vi "joysticki.vi"(9 "Multicolumn Listbox":i32(listbox), 10 "stop":bool) -> (11 "Numeric":i32)   [LabVIEW 2015]
uses:
  <vilib>/MakerHub/Xbox-One-Controller/Private/Type Defs/Xbox Controller Device.ctl
  <vilib>/Utility/inputDevices.llb/closeJoystick.vi
  <vilib>/MakerHub/Xbox-One-Controller/LMH-Xbox-One-Controller.lvlib
panel:
  out "output cluster":T1
  out "mouse info":T2(array[cluster])
  out "key info":T3(array[cluster])
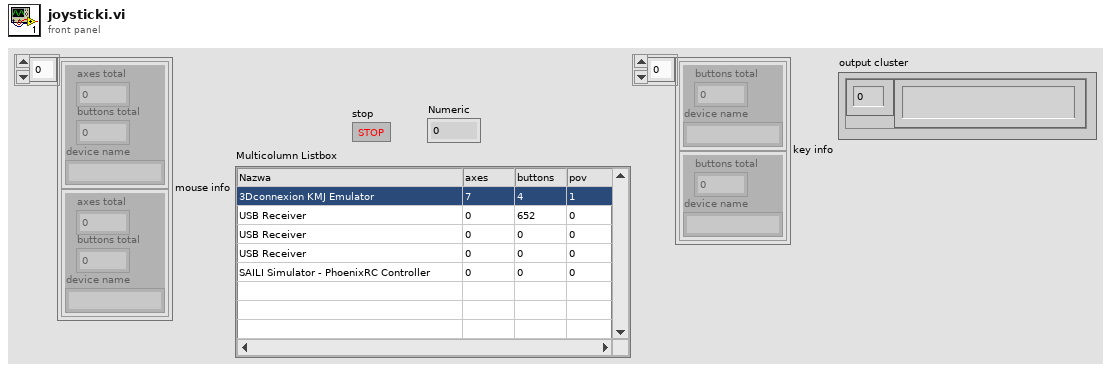
[diagram p1: front panel]
types:
  T1 = typedef "LMH-Xbox-One-Controller.lvlib/Xbox Controller Device.ctl" = cluster{"Device Index":i32, "Device Name":string}
  T2 = cluster{"axes total":u32, "buttons total":u32, "device name":string}[]
  T3 = cluster{"buttons total":u32, "device name":string}[]
  T4 = cluster{"axes total":u32, "buttons total":u32, "pov total":u32, "device name":string}[]
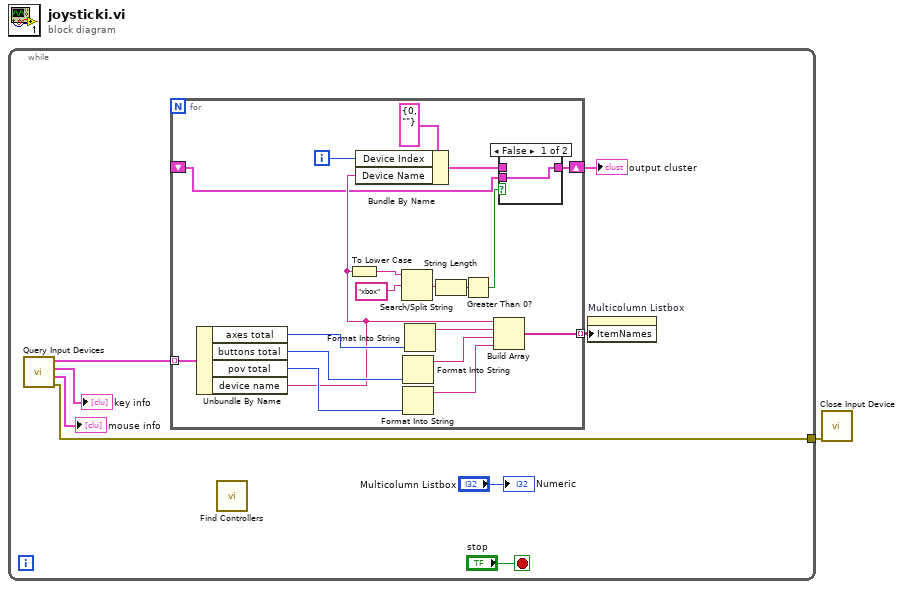
[diagram p0: block diagram]
diagram:
  n1 = while {
    tunnel: [w3] -> w1
    stop <- "stop" stop-if-true
    n2 = call <vilib>:"Query Input Devices.vi"() -> ("error out"=w3:errorcluster, "mouse info"=→"mouse info":T2, "key info"=→"key info":T3, "joystick info"=w9:T4)  [unwired: 8 in]
    n3 = for {
      tunnel: w9 -> [w21] mode=indexing
      tunnel: [w28] -> w7 mode=indexing
      shift-right: [w18] -> w2
      shift-left: _ -> [w10]
      i -> [w16]
      n4 = Unbundle By Name(w21) -> ("axes total"=w22:u32, "buttons total"=w26:u32, "pov total"=w25:u32, "device name"=w19:string)
      n5 = To Lower Case(string=w19) -> (all lower case string=w15:string)
      n6 = Bundle By Name(cluster=T1 {"Device Index"=0, "Device Name"=""} ("Xbox Controllers"), "Device Index"=w16, "Device Name"=w19) -> (w17:T1)
      n7 = Search/Split String(string=w15, search string/char (-)="xbox") -> (match + rest of string=w13:string)  [unwired: 1 in, 2 out]
      n8 = Format Into String(w26) -> (resulting string=w24:string)  [unwired: 3 in, 1 out]
      n9 = Format Into String(w25) -> (resulting string=w23:string)  [unwired: 3 in, 1 out]
      n10 = Format Into String(w22) -> (resulting string=w27:string)  [unwired: 3 in, 1 out]
      n11 = String Length(string=w13) -> (length=w12:i32)
      n12 = Greater Than 0?(x=w12) -> (x > 0?=w11:bool)
      n13 = Build Array(w19, w27, w24, w23) -> (w28:string[])
      n14 = case shown="False" w11 {
        tunnel: [w29 w30] -> w18
        tunnel: w17 -> [_ w30]
        tunnel: w10 -> [w29 _]
        frame False {
        }
        frame True {
        }
      }
    }
    "output cluster" <- w2
    n15 = call <vilib>:"Find Controllers.vi"() -> ()  [unwired: 10 in, 2 out]
    n16 = property on="Multicolumn Listbox" class="MCListbox (strict)"("ItemNames"=w7) -> ()  [unwired: 2 in, 2 out]
    "Numeric" <- "Multicolumn Listbox"
  }
  n17 = call-poly <vilib>:"Close Input Device.vi"("error in (no error)"=w1) -> ()  [unwired: 9 in, 1 out]
